vi "Init Module.vi"(8 "error in":errorcluster, 11 "Singleton Module Admin in":refnum<class "Delacor_lib_QMH_Module Admin.lvclass">) -> (0 "error out":errorcluster, 2 "Analysis Request Events":T1, 3 "Singleton Module Admin out":refnum<class "Delacor_lib_QMH_Module Admin.lvclass">)   [LabVIEW 2019, in "Analysis.lvlib"]
doc: "Initialize the module by creating Broadcast Events, Request Events, and synchronization rendezvous.\n_____\nBased on Delacor QMH Project Template 4.0.0.47.\n_____\nBased on DQMH Project Template 6.1.0.94."
uses:
  Analysis.lvlib
  <vilib>/Delacor/Delacor QMH/Libraries/Module Admin_class/Delacor_lib_QMH_Module Admin.lvclass
  Request Events--cluster.ctl
  Stop Argument--cluster.ctl
  Show Panel Argument--cluster.ctl
  Hide Panel Argument--cluster.ctl
  Get Module Execution Status Argument--cluster.ctl
  Show Diagram Argument--cluster.ctl
  Wakeup Helper Loop Argument--cluster.ctl
  Change Settings Argument--cluster.ctl
  Main UI Shared/Signal Type--enum.ctl
  Main UI Shared/Calibration Values--cluster.ctl
  Update analysis parameters Argument--cluster.ctl
  Main UI Shared/Decimation input --cluster.ctl
  Update analysis parameters (Reply Payload)--cluster.ctl
  Update Savitzky parameters Argument--cluster.ctl
  Update decimation Argument--cluster.ctl
  Update contact parameters Argument--cluster.ctl
  Update Tau delay (ms) Argument--cluster.ctl
  Open Fcurve object Argument--cluster.ctl
  Neo-Laura-LVOOP/SignalViewer/TDMS_DataHandler_class/Fcurve Meta data.ctl
  Open Fcurve object (Reply Payload)--cluster.ctl
  Neo-Laura-LVOOP/Class Library/Fcurve_class/Metadata.ctl
  Main UI Shared/MAIN UI Shared.lvlib
  Neo-Laura-LVOOP/SignalViewer/TDMS_DataHandler_class/TDMS_DataHandler.lvclass
  Neo-Laura-LVOOP/Class Library/Fcurve_class/Fcurve.lvclass
panel:
  # "Contact"
  # "Contact"
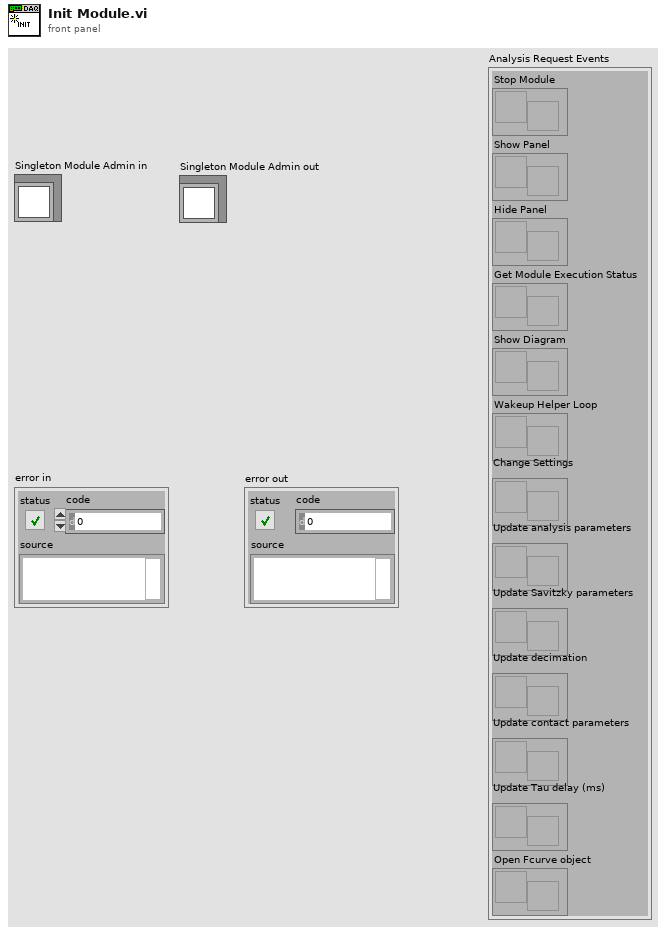
[diagram p1: front panel]
types:
  T1 = typedef "Analysis.lvlib/Request Events--cluster.ctl" = cluster{"Stop Module":refnum<user-event>, "Show Panel":refnum<user-event>, "Hide Panel":refnum<user-event>, "Get Module Execution Status":refnum<user-event>, "Show Diagram":refnum<user-event>, "Wakeup Helper Loop":refnum<user-event>, "Change Settings":refnum<user-event>, "Update analysis parameters":refnum<user-event>, "Update Savitzky parameters":refnum<user-event>, "Update decimation":refnum<user-event>, "Update contact parameters":refnum<user-event>, "Update Tau delay (ms)":refnum<user-event>, "Open Fcurve object":refnum<user-event>}
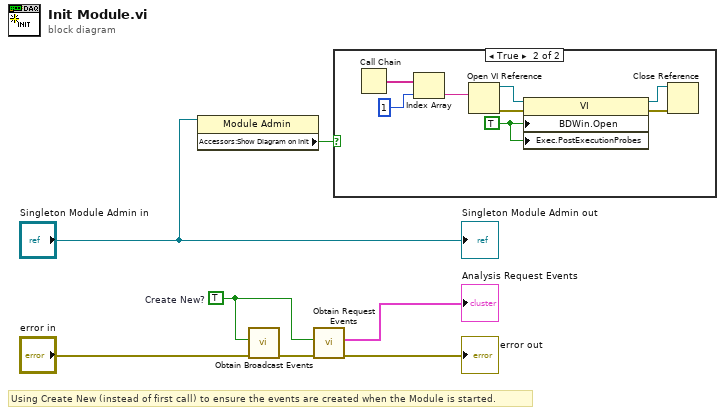
[diagram p0: block diagram]
diagram:
  w4 = TRUE  # Create New?
  # "Using Create New (instead of first call) to ensure the events are created when the Module is started."
  n1 = property class="Module Admin"(reference="Singleton Module Admin in") -> ("Accessors:Show Diagram on Init"=w2:bool)  [unwired: 1 in, 2 out]
  n2 = call "Obtain Broadcast Events.vi"("error in (no error)"="error in", "Create New? (F)"=w4) -> ("error out"=w7:errorcluster)  [unwired: 8 in, 1 out]
  n3 = call "Obtain Request Events.vi"("error in (no error)"=w7, "Create New? (F)"=w4) -> ("error out"=→"error out":errorcluster, "Analysis Request Events"=→"Analysis Request Events":T1)  [unwired: 8 in]
  n4 = case shown="True" w2 {
    frame False {
    }
    frame True {
      w11 = TRUE ("Block Diagram Window:Open")
      n5 = Call Chain() -> (call chain=w15:string[])
      n6 = Index Array(array=w15, index=1) -> (element=w8:string)
      n7 = Open VI Reference(vi path=w8) -> (vi reference=w12:refnum<vi>, error out=w13:errorcluster)  [unwired: 5 in]
      n8 = property class="VI"(reference=w12, error in=w13, "BDWin.Open"=w11, "Exec.PostExecutionProbes"=w11) -> (reference out=w9:refnum<vi>, error out=w10:errorcluster)
      n9 = Close Reference(reference=w9, error in (no error)=w10) -> ()  [unwired: 1 out]
    }
  }
  "Singleton Module Admin out" <- "Singleton Module Admin in"
